vi "Stop Core.vi"(10 "final error code":i32, 11 "Actor in":refnum<class "Actor1_Basic_N_4.0.0.lvclass">) -> (3 "Actor out":refnum<class "Actor1_Basic_N_4.0.0.lvclass">)   [LabVIEW 2020, in "Actor1_Basic_N_4.0.0.lvlib" / "Actor1_Basic_N_4.0.0.lvclass"]
uses:
  Actor1_Basic_N_4.0.0.lvclass
  <vilib>/ActorFramework/Actor/Actor.lvclass
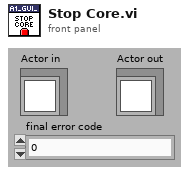
[diagram p1: front panel]
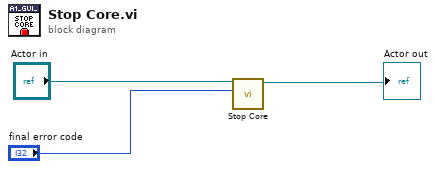
[diagram p0: block diagram]
diagram:
  n1 = call-parent "Stop Core.vi"("final error code"="final error code", "Actor in"="Actor in") -> ("Actor out"=→"Actor out":refnum<class "Actor1_Basic_N_4.0.0.lvclass">)  [unwired: 9 in]
